vi "Create Function String (Motor).vi"(8 "error in (no error)":errorcluster, 9 "Element/Wiring Unit (1: 1)":i32(ring)=1 items=["Null", "1", "2", "3", "4", "5", "6", "Sigma A", "Sigma B", "Sigma C"], 10 "Function (0: Speed)":i32(ring) items=["Speed", "Torque", "Synchronize Sp", "Slip", "Pm", "EaU", "EaI"], 11 "VISA resource name":refnum<visa-resource-name>) -> (0 "error out":errorcluster, 2 "Function String":string, 3 "VISA resource name out":refnum<visa-resource-name>)   [LabVIEW 2021, in "Yokogawa WT1800 Series.lvlib"]
doc: "Create a motor function string.\n\n<b>Note:</b>\nThis setting valid on models with the motor evaluation function (/MTR) option."
uses:
  <instrlib>/Yokogawa WT1800 Series/Yokogawa WT1800 Series.lvlib
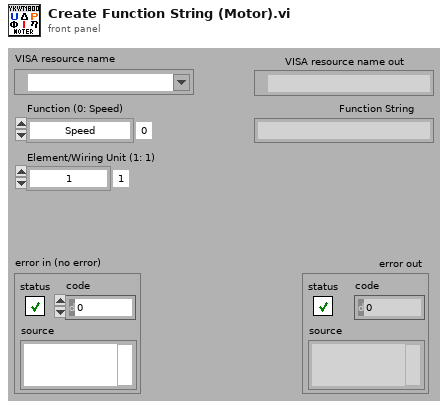
[diagram p1: front panel]
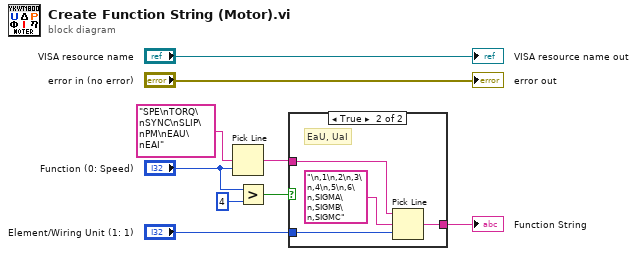
[diagram p0: block diagram]
diagram:
  n1 = Pick Line ("ライン選択")(multi-line string="SPE\nTORQ\nSYNC\nSLIP\nPM\nEAU\nEAI" ("複数行文字列"), line index="Function (0: Speed)") -> (output string=w7:string)  [unwired: 1 in]
  n2 = Greater?(x="Function (0: Speed)", y=4) -> (0:w3:bool)
  n3 = case shown="True" w3 {
    tunnel: w7 -> [w10 w13]
    tunnel: "Element/Wiring Unit (1: 1)" -> [_ w12]
    tunnel: [w10 w11] -> w4
    frame False {
      # "Not EAU, EAI"
    }
    frame True {
      # "EaU, UaI"
      n4 = Pick Line ("ライン選択")(string ("")=w13, multi-line string="\n,1\n,2\n,3\n,4\n,5\n,6\n,SIGMA\n,SIGMB\n,SIGMC" ("複数行文字列"), line index=w12) -> (output string=w11:string)
    }
  }
  "Function String" <- w4
  "VISA resource name out" <- "VISA resource name"
  "error out" <- "error in (no error)"
